vi "Engine Out - GDI - Boost Actuation.vi"(10 "Wastegate Position Setpoint [%Open]":sgl, 11 "TurboBPV Position Setpoint [%Open]":sgl) -> (2 "Wastegate LS Output":T1, 3 "TurboBPV LS Output":T1)   [LabVIEW 2015, in "ECS-RT.lvlib"]
uses:
  ECS-RT.lvlib
  Typedefs/Raw Outputs/LS.ctl
  ECS-Shared.lvlib
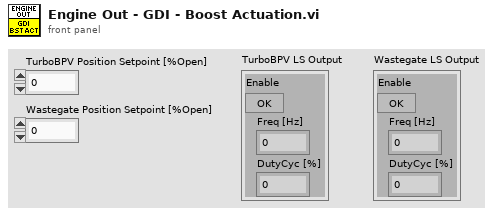
[diagram p1: front panel]
types:
  T1 = typedef "ECS-Shared.lvlib/LS.ctl" = cluster{"Enable":bool, "Freq [Hz]":sgl, "DutyCyc [%]":sgl}
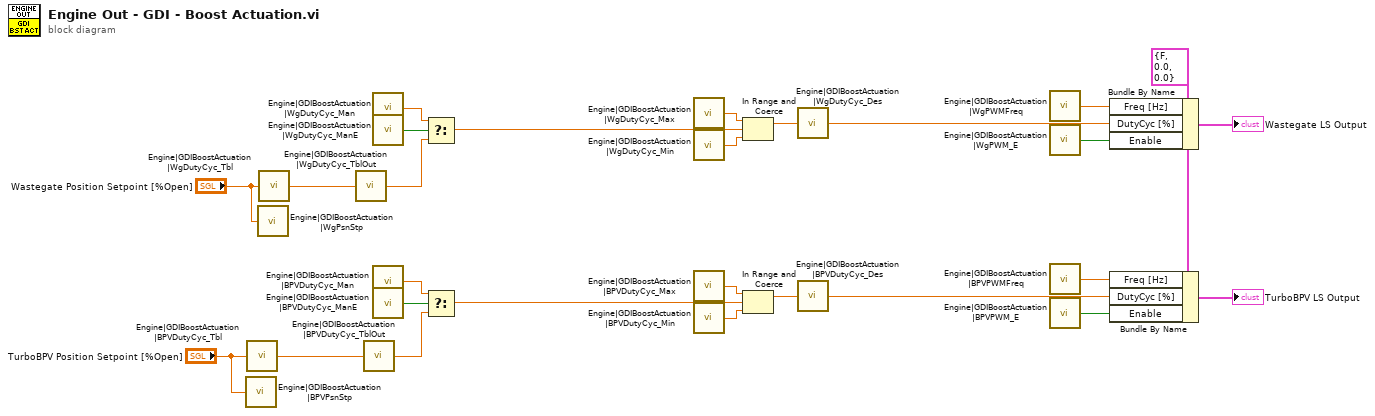
[diagram p0: block diagram]
diagram:
  w9 = T1 {"Enable"=FALSE, "Freq [Hz]"=0.0, "DutyCyc [%]"=0.0} ("LS Output")
  n1 = call "Engine|GDIBoostActuation|BPVPsnStp"("Value"="TurboBPV Position Setpoint [%Open]") -> ()
  n2 = call "Engine|GDIBoostActuation|BPVDutyCyc_Tbl"("X Index"="TurboBPV Position Setpoint [%Open]") -> ("Y"=w4:sgl)
  n3 = call "Engine|GDIBoostActuation|WgPsnStp"("Value"="Wastegate Position Setpoint [%Open]") -> ()
  n4 = call "Engine|GDIBoostActuation|WgDutyCyc_Tbl"("X Index"="Wastegate Position Setpoint [%Open]") -> ("Y"=w3:sgl)
  n5 = call "Engine|GDIBoostActuation|WgDutyCyc_TblOut"("Value"=w3) -> ()
  n6 = call "Engine|GDIBoostActuation|BPVDutyCyc_TblOut"("Value"=w4) -> ()
  n7 = call "Engine|GDIBoostActuation|WgDutyCyc_Man"() -> ("Value"=w13:sgl)
  n8 = call "Engine|GDIBoostActuation|WgDutyCyc_ManE"() -> ("Value"=w14:bool)
  n9 = call "Engine|GDIBoostActuation|BPVDutyCyc_Man"() -> ("Value"=w12:sgl)
  n10 = call "Engine|GDIBoostActuation|BPVDutyCyc_ManE"() -> ("Value"=w11:bool)
  n11 = Select(t=w13, s=w14, f=w3) -> (s? t:f=w15:sgl)
  n12 = Select(t=w12, s=w11, f=w4) -> (s? t:f=w10:sgl)
  n13 = call "Engine|GDIBoostActuation|WgDutyCyc_Max"() -> ("Value"=w16:sgl)
  n14 = call "Engine|GDIBoostActuation|WgDutyCyc_Min"() -> ("Value"=w17:sgl)
  n15 = call "Engine|GDIBoostActuation|BPVDutyCyc_Max"() -> ("Value"=w18:sgl)
  n16 = call "Engine|GDIBoostActuation|BPVDutyCyc_Min"() -> ("Value"=w19:sgl)
  n17 = In Range and Coerce(upper limit=w16, x=w15, lower limit=w17) -> (coerced(x)=w2:sgl)  [unwired: 1 out]
  n18 = In Range and Coerce(upper limit=w18, x=w10, lower limit=w19) -> (coerced(x)=w1:sgl)  [unwired: 1 out]
  n19 = call "Engine|GDIBoostActuation|WgDutyCyc_Des"("Value"=w2) -> ()
  n20 = call "Engine|GDIBoostActuation|BPVDutyCyc_Des"("Value"=w1) -> ()
  n21 = call "Engine|GDIBoostActuation|WgPWMFreq"() -> ("Value"=w22:sgl)
  n22 = call "Engine|GDIBoostActuation|WgPWM_E"() -> ("Value"=w21:bool)
  n23 = call "Engine|GDIBoostActuation|BPVPWMFreq"() -> ("Value"=w23:sgl)
  n24 = call "Engine|GDIBoostActuation|BPVPWM_E"() -> ("Value"=w20:bool)
  n25 = Bundle By Name(cluster=w9, "Freq [Hz]"=w22, "DutyCyc [%]"=w2, "Enable"=w21) -> (→"Wastegate LS Output":T1)
  n26 = Bundle By Name(cluster=w9, "Freq [Hz]"=w23, "DutyCyc [%]"=w1, "Enable"=w20) -> (→"TurboBPV LS Output":T1)
